vi "1553B_Msg_cirle.vi"(7 "Timeout(默认:5ms)":i32=5, 8 "error in":errorcluster, 10 "主备份选择":enum8{"主份", "备份"}(ring), 11 "VISA资源名称":refnum<visa-resource-name>) -> (0 "error out 2":errorcluster, 1 "timeout":bool, 3 "VISAout":refnum<visa-resource-name>)   [LabVIEW 2012]
uses:
  <vilib>/GPower/VIRegister/Library/Convert/ToU32.vi
  <vilib>/GPower/VIRegister/Library/Convert/ToU8.vi
  <vilib>/GPower/VIRegister/Library/SubVIs/FindRegisterData.vi
  <vilib>/GPower/VIRegister/Library/SubVIs/ReadSub.vi
  <vilib>/GPower/VIRegister/Library/QManager/GetRegisterData.vi
  <vilib>/GPower/Error/Library/SetError.vi
  <vilib>/GPower/Error/Library/FilterCodes.vi
  <vilib>/GPower/Error/Library/Filter/FilterMulti.vi
  <vilib>/GPower/VIRegister/Library/QManager/QManagerAction.vi
  <vilib>/GPower/Error/Library/ErrorType.vi
  <vilib>/GPower/Error/Library/SplitAppended.vi
  <vilib>/GPower/Error/Library/SubVIs/ExplanationToError.vi
  com/TONGXUN/write32.vi
  com/TONGXUN/write8.vi
  <vilib>/GPower/VIRegister/Library/QManager/GetQName.vi
  <vilib>/GPower/VIRegister/Library/QManager/StartQManager.vi
  <vilib>/Utility/error.llb/Trim Whitespace.vi
  <vilib>/dlg_ctls.llb/Space Constant.vi
  <vilib>/Utility/error.llb/Error Code Database.vi
  <vilib>/GPower/Error/Library/SubVIs/SetStatus.vi
  <vilib>/GPower/Error/Library/AppendErrors.vi
  <vilib>/GPower/Error/Library/Append/AppendSingle.vi
  <vilib>/GPower/VIRegister/VIRegister.lvlib
panel:
  out "x+y 4":u32 format="%.0x"
  out "timeout 2":bool
  out "x+y 2":u32 format="%.0x"
  out "x+y":u32 format="%.0x"
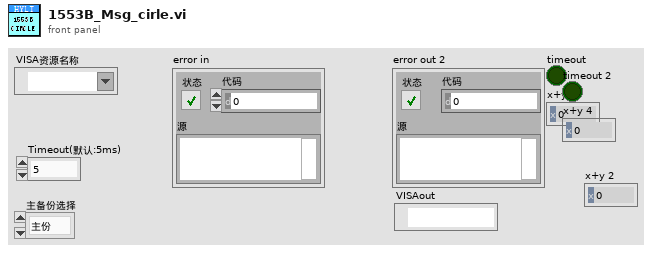
[diagram p1: front panel]
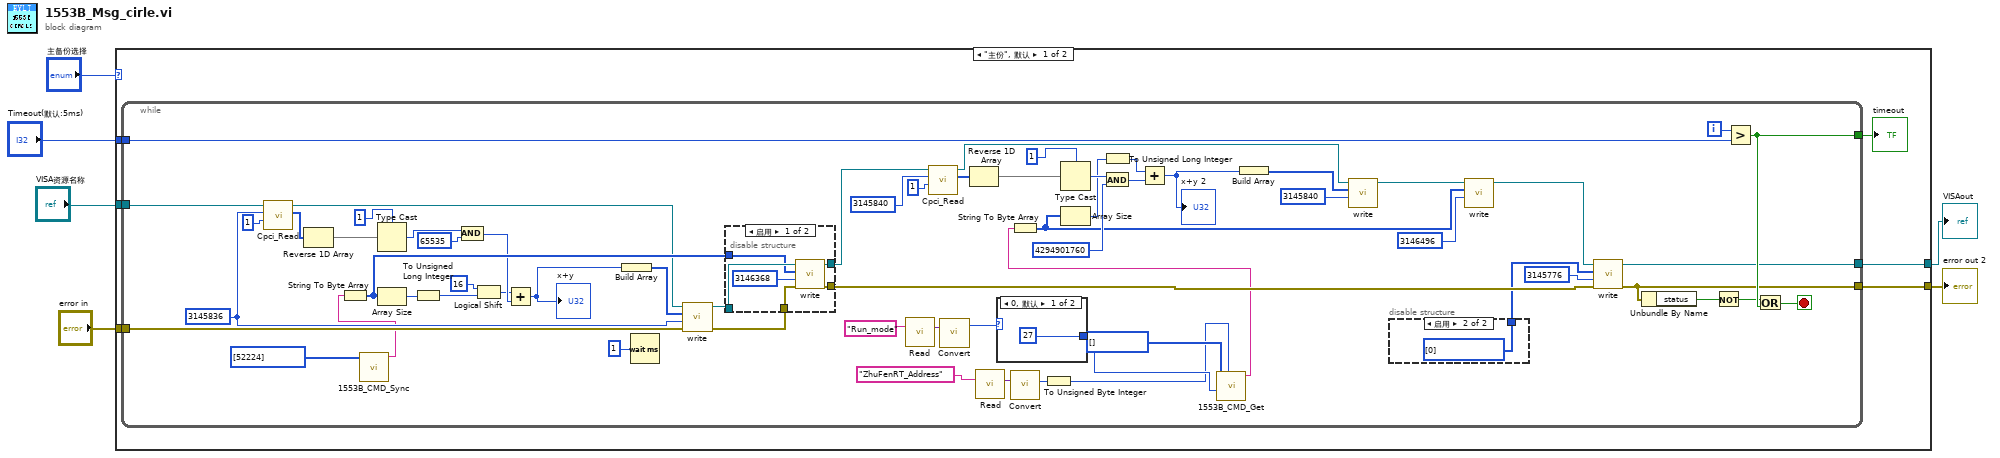
[diagram p0: block diagram]
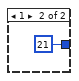
[diagram p3: hidden frame]
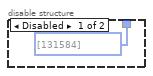
[diagram p4: hidden frame]
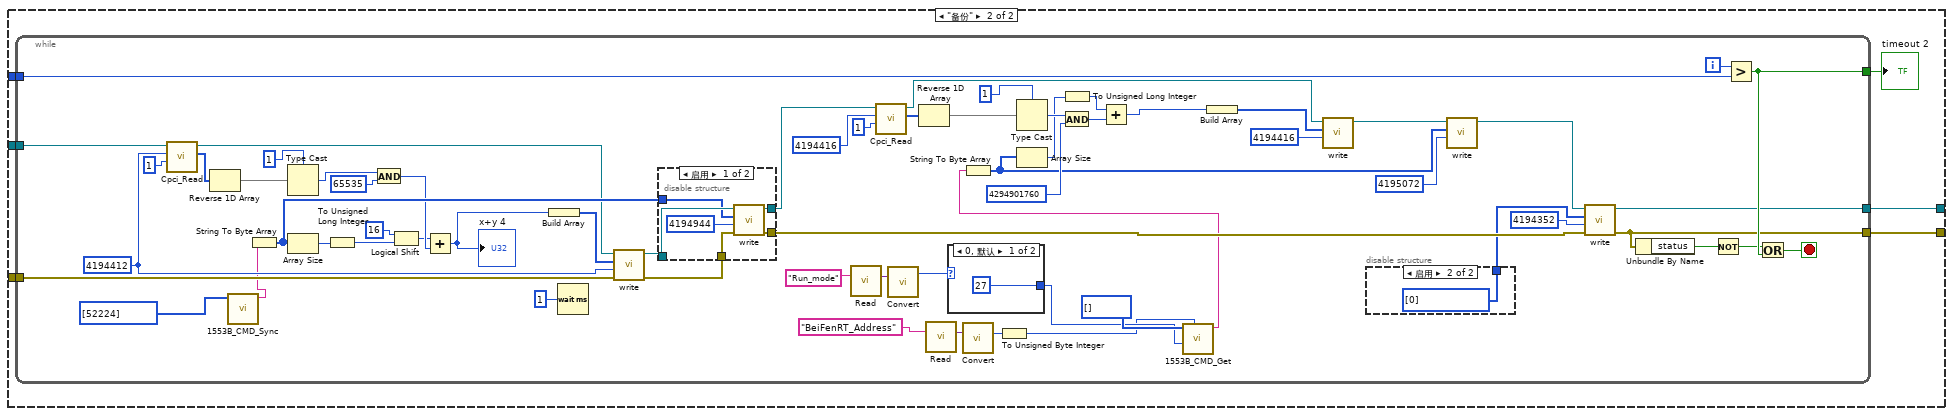
[diagram p5: hidden frame]
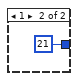
[diagram p7: hidden frame]
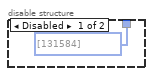
[diagram p8: hidden frame]
diagram:
  n1 = case shown="\"主份\", 默认" "主备份选择" {
    tunnel: "Timeout(默认:5ms)" -> [w11 w92]
    tunnel: "error in" -> [w10 w91]
    tunnel: [w9 w90] -> w3
    tunnel: [w8 w89] -> w2
    tunnel: "VISA资源名称" -> [w7 w88]
    frame "主份", Default {
      n2 = while {
        tunnel: w7 -> [w59]
        tunnel: w10 -> [w75]
        tunnel: [w63] -> w9
        tunnel: [w71] -> w12
        tunnel: [w70] -> w8
        tunnel: w11 -> [w24]
        i -> [w73]
        stop <- w72 stop-if-true
        w58 = u32 3145836 ("偏移量(0)")
        n3 = call "Cpci_Read.vi"("u32_len"=1, "基地址"=w58, "VISA资源名称"=w59) -> ("U8"=w26:u8[], "VISA资源名称输出"=w56:refnum<visa-resource-name>)  [unwired: 6 in, 1 out]
        n4 = Reverse 1D Array(array=w26) -> (reversed array=w25:u8[])
        n5 = call "1553B_CMD_Sync.vi"("数据字数组"=u16[] [52224]) -> ("1553B指令"=w13:string)  [unwired: 10 in]
        n6 = String To Byte Array(string=w13) -> (unsigned byte array=w60:u8[])
        n7 = Type Cast(type=u32 1 ("u32_len"), x=w25) -> (*(type *) &x=w53:u32)
        n8 = Array Size(array=w60) -> (size(s)=w69:i32)
        n9 = To Unsigned Long Integer(number=w69) -> (unsigned 32bit integer=w51:u32)
        n10 = And(x=w53, y=u32 65535) -> (x .and. y?=w52:u32)
        n11 = Logical Shift(y=i16 16, x=w51) -> (x << y=w49:u32)
        n12 = Add(x=w49, y=w52) -> (x+y=w50:u32)
        "x+y" <- w50
        n13 = Build Array(w50) -> (w68:u32[])
        n14 = Wait (ms)(milliseconds to wait=u32 1 ("等待时间（毫秒）")) -> ()  [unwired: 1 out]
        n15 = call-poly "write.vi"("error out"=w75, "起始地址"=w58, "U32"=w68, "VISA资源名称输入"=w56) -> ("error out 2"=w66:errorcluster, "VISA资源名称输出"=w64:refnum<visa-resource-name>)  [unwired: 6 in]
        n16 = disable-structure shown="启用" {
          disable-tunnel: w66 -> [w80 w82]
          disable-tunnel: [w79 w82] -> w65
          disable-tunnel: w64 -> [w78 w83]
          disable-tunnel: w60 -> [w77 _]
          disable-tunnel: [w76 w83] -> w42
          frame Enabled {
            n17 = call-poly "write.vi"("error out"=w80, "起始地址"=u32 3146368 ("偏移量(0)"), "数组"=w77, "VISA资源名称输入"=w78) -> ("error out 2"=w79:errorcluster, "VISA资源名称 输出"=w76:refnum<visa-resource-name>)  [unwired: 6 in]
          }
          frame Disabled {
          }
        }
        n18 = call <vilib>:"Read.vi"("Register name"="Run_mode") -> ("Register value"=w21:variant)  [unwired: 11 in, 3 out]
        n19 = call "Cpci_Read.vi"("u32_len"=1, "基地址"=u32 3145840 ("偏移量(0)"), "VISA资源名称"=w42) -> ("U8"=w36:u8[], "VISA资源名称输出"=w29:refnum<visa-resource-name>)  [unwired: 6 in, 1 out]
        n20 = call-poly <vilib>:"Convert.vi"("Register value in"=w21) -> ("Register value out"=w20:u8)  [unwired: 13 in, 1 out]
        n21 = Reverse 1D Array(array=w36) -> (reversed array=w37:u8[])
        n22 = call <vilib>:"Read.vi"("Register name"="ZhuFenRT_Address") -> ("Register value"=w17:variant)  [unwired: 11 in, 3 out]
        n23 = case shown="0, 默认" w20 {
          tunnel: [u16 27 ("字长") u16 21 ("字长")] -> w19
          frame 0, Default {
          }
          frame 1 {
          }
        }
        n24 = call-poly <vilib>:"Convert.vi"("Register value in"=w17) -> ("Register value out"=w16:u32)  [unwired: 13 in, 1 out]
        n25 = To Unsigned Byte Integer(number=w16) -> (unsigned 8bit integer=w15:u8)
        n26 = Type Cast(type=u32 1 ("u32_len"), x=w37) -> (*(type *) &x=w40:u32)
        n27 = And(x=w40, y=u32 4294901760) -> (x .and. y?=w35:u32)
        n28 = call "1553B_CMD_Get.vi"("RT地址(默认：01111)"=w15, "字长"=w19, "数据字数组"=u16[] []) -> ("1553B指令"=w46:string)  [unwired: 8 in]
        n29 = String To Byte Array(string=w46) -> (unsigned byte array=w33:u8[])
        n30 = Array Size(array=w33) -> (size(s)=w34:i32)
        n31 = To Unsigned Long Integer(number=w34) -> (unsigned 32bit integer=w32:u32)
        n32 = Add(x=w32, y=w35) -> (x+y=w31:u32)
        "x+y 2" <- w31
        n33 = Build Array(w31) -> (w30:u32[])
        n34 = call-poly "write.vi"("起始地址"=u32 3145840 ("偏移量(0)"), "U32"=w30, "VISA资源名称输入"=w29) -> ("VISA资源名称输出"=w27:refnum<visa-resource-name>)  [unwired: 7 in, 1 out]
        n35 = disable-structure shown="启用" {
          disable-tunnel: [u32[] [131584] ("U32") u32[] [0] ("U32")] -> w23
          frame Disabled {
          }
          frame Enabled {
          }
        }
        n36 = call-poly "write.vi"("起始地址"=u32 3146496, "数组"=w33, "VISA资源名称输入"=w27) -> ("VISA资源名称 输出"=w44:refnum<visa-resource-name>)  [unwired: 7 in, 1 out]
        n37 = call-poly "write.vi"("error out"=w65, "起始地址"=u32 3145776 ("偏移量(0)"), "U32"=w23, "VISA资源名称输入"=w44) -> ("error out 2"=w63:errorcluster, "VISA资源名称输出"=w70:refnum<visa-resource-name>)  [unwired: 6 in]
        n38 = Unbundle By Name(w63) -> ("status"=w62:bool)
        n39 = Not(x=w62) -> (.not. x?=w61:bool)
        n40 = Greater?(x=w73, y=w24) -> (0:w71:bool)
        n41 = Or(x=w61, y=w71) -> (x .or. y?=w72:bool)
      }
      "timeout" <- w12
    }
    frame "备份" {
      n42 = while {
        tunnel: w88 -> [w140]
        tunnel: w91 -> [w156]
        tunnel: [w144] -> w90
        tunnel: [w152] -> w93
        tunnel: [w151] -> w89
        tunnel: w92 -> [w105]
        i -> [w154]
        stop <- w153 stop-if-true
        w139 = u32 4194412 ("偏移量(0)")
        n43 = call "Cpci_Read.vi"("u32_len"=1, "基地址"=w139, "VISA资源名称"=w140) -> ("U8"=w107:u8[], "VISA资源名称输出"=w137:refnum<visa-resource-name>)  [unwired: 6 in, 1 out]
        n44 = Reverse 1D Array(array=w107) -> (reversed array=w106:u8[])
        n45 = call "1553B_CMD_Sync.vi"("数据字数组"=u16[] [52224]) -> ("1553B指令"=w98:string)  [unwired: 10 in]
        n46 = String To Byte Array(string=w98) -> (unsigned byte array=w141:u8[])
        n47 = Type Cast(type=u32 1 ("u32_len"), x=w106) -> (*(type *) &x=w134:u32)
        n48 = Array Size(array=w141) -> (size(s)=w150:i32)
        n49 = To Unsigned Long Integer(number=w150) -> (unsigned 32bit integer=w132:u32)
        n50 = And(x=w134, y=u32 65535) -> (x .and. y?=w133:u32)
        n51 = Logical Shift(y=i16 16, x=w132) -> (x << y=w130:u32)
        n52 = Add(x=w130, y=w133) -> (x+y=w131:u32)
        "x+y 4" <- w131
        n53 = Build Array(w131) -> (w149:u32[])
        n54 = Wait (ms)(milliseconds to wait=u32 1 ("等待时间（毫秒）")) -> ()  [unwired: 1 out]
        n55 = call-poly "write.vi"("error out"=w156, "起始地址"=w139, "U32"=w149, "VISA资源名称输入"=w137) -> ("error out 2"=w147:errorcluster, "VISA资源名称输出"=w145:refnum<visa-resource-name>)  [unwired: 6 in]
        n56 = disable-structure shown="启用" {
          disable-tunnel: w147 -> [w161 w163]
          disable-tunnel: [w160 w163] -> w146
          disable-tunnel: w145 -> [w159 w164]
          disable-tunnel: w141 -> [w158 _]
          disable-tunnel: [w157 w164] -> w123
          frame Enabled {
            n57 = call-poly "write.vi"("error out"=w161, "起始地址"=u32 4194944 ("偏移量(0)"), "数组"=w158, "VISA资源名称输入"=w159) -> ("error out 2"=w160:errorcluster, "VISA资源名称 输出"=w157:refnum<visa-resource-name>)  [unwired: 6 in]
          }
          frame Disabled {
          }
        }
        n58 = call <vilib>:"Read.vi"("Register name"="Run_mode") -> ("Register value"=w102:variant)  [unwired: 11 in, 3 out]
        n59 = call "Cpci_Read.vi"("u32_len"=1, "基地址"=u32 4194416 ("偏移量(0)"), "VISA资源名称"=w123) -> ("U8"=w117:u8[], "VISA资源名称输出"=w110:refnum<visa-resource-name>)  [unwired: 6 in, 1 out]
        n60 = call-poly <vilib>:"Convert.vi"("Register value in"=w102) -> ("Register value out"=w101:u8)  [unwired: 13 in, 1 out]
        n61 = Reverse 1D Array(array=w117) -> (reversed array=w118:u8[])
        n62 = call <vilib>:"Read.vi"("Register name"="BeiFenRT_Address") -> ("Register value"=w96:variant)  [unwired: 11 in, 3 out]
        n63 = case shown="0, 默认" w101 {
          tunnel: [u16 27 ("字长") u16 21 ("字长")] -> w100
          frame 0, Default {
          }
          frame 1 {
          }
        }
        n64 = call-poly <vilib>:"Convert.vi"("Register value in"=w96) -> ("Register value out"=w95:u32)  [unwired: 13 in, 1 out]
        n65 = To Unsigned Byte Integer(number=w95) -> (unsigned 8bit integer=w94:u8)
        n66 = Type Cast(type=u32 1 ("u32_len"), x=w118) -> (*(type *) &x=w121:u32)
        n67 = And(x=w121, y=u32 4294901760) -> (x .and. y?=w116:u32)
        n68 = call "1553B_CMD_Get.vi"("RT地址(默认：01111)"=w94, "字长"=w100, "数据字数组"=u16[] []) -> ("1553B指令"=w127:string)  [unwired: 8 in]
        n69 = String To Byte Array(string=w127) -> (unsigned byte array=w114:u8[])
        n70 = Array Size(array=w114) -> (size(s)=w115:i32)
        n71 = To Unsigned Long Integer(number=w115) -> (unsigned 32bit integer=w113:u32)
        n72 = Add(x=w113, y=w116) -> (x+y=w112:u32)
        n73 = Build Array(w112) -> (w111:u32[])
        n74 = call-poly "write.vi"("起始地址"=u32 4194416 ("偏移量(0)"), "U32"=w111, "VISA资源名称输入"=w110) -> ("VISA资源名称输出"=w108:refnum<visa-resource-name>)  [unwired: 7 in, 1 out]
        n75 = disable-structure shown="启用" {
          disable-tunnel: [u32[] [131584] ("U32") u32[] [0] ("U32")] -> w104
          frame Disabled {
          }
          frame Enabled {
          }
        }
        n76 = call-poly "write.vi"("起始地址"=u32 4195072, "数组"=w114, "VISA资源名称输入"=w108) -> ("VISA资源名称 输出"=w125:refnum<visa-resource-name>)  [unwired: 7 in, 1 out]
        n77 = call-poly "write.vi"("error out"=w146, "起始地址"=u32 4194352 ("偏移量(0)"), "U32"=w104, "VISA资源名称输入"=w125) -> ("error out 2"=w144:errorcluster, "VISA资源名称输出"=w151:refnum<visa-resource-name>)  [unwired: 6 in]
        n78 = Unbundle By Name(w144) -> ("status"=w143:bool)
        n79 = Not(x=w143) -> (.not. x?=w142:bool)
        n80 = Greater?(x=w154, y=w105) -> (0:w152:bool)
        n81 = Or(x=w142, y=w152) -> (x .or. y?=w153:bool)
      }
      "timeout 2" <- w93
    }
  }
  "error out 2" <- w3
  "VISAout" <- w2
